vi "Status of Migration.vi"(7 "Pass?T":bool) -> (3 "Status":string)   [LabVIEW 2021, in "Error Logger.lvlib"]
uses:
  Error Logger.lvlib
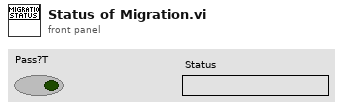
[diagram p1: front panel]
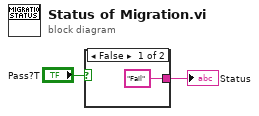
[diagram p0: block diagram]
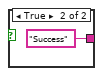
[diagram p2: hidden frame]
diagram:
  n1 = case shown="False" "Pass?T" {
    tunnel: ["Fail" "Success"] -> w1
    frame False {
    }
    frame True {
    }
  }
  "Status" <- w1
